vi "Process.vi"(8 "error in":errorcluster, 11 "LHF.SimpleAuth.User":refnum<class "LHF.SimpleAuth.User.lvclass">) -> (0 "error out":errorcluster={"status"=TRUE, "code"=1556, "source"="In Place Element Structure in SMO.lvclass:GetProtectedEvents.vi->SMO.lvclass:Process.vi:5310001->SMO.UI.lvclass:Process.vi:5310001->LHF.SimpleAuth.User.lvclass:Process.vi"}, 3 "LHF.SimpleAuth.User out":refnum<class "LHF.SimpleAuth.User.lvclass">)   [LabVIEW 2013, in "LHF.SimpleAuth.User.lvclass"]
doc: "---------------------------------------------------------------\nJKI State Machine Objects™\nhttp://jki.net/state-machine-objects/\nCopyright (C) 2005-2015, JKI <info@jki.net>\nALL RIGHTS RESERVEDJKI State Machine Objects (SMO) 1.0.0.5\nJKI - JKI\nCopyright (c) 2016, JKI"
uses:
  LHF.SimpleAuth.User.lvclass
  <vilib>/JKI/JKI SMO/SMO/Typedefs/Parent Call--Enum.ctl
  <vilib>/JKI/JKI SMO/SMO.UI/SMO.UI.lvclass
  <userlib>/LHF/MongoDB/LHF.DB.Mongo.lvclass
  <userlib>/_OpenG.lib/md5/md5.llb/MD5 Message Digest (Hexadecimal String)__ogtk.vi
  <vilib>/JKI/JKI SMO/SMO/SMO.lvclass
panel:
  in  "Action: Edit >> Level":T1(ring)
  in  "Action: Edit >> Name":string
  in  "Action: Edit >> Login":string
  in  "Action: Load User":i32(listbox)=-1
  in  "Action: Save":bool
  in  "Action: Set Password":bool
  in  "Action: Remove":bool
  # "For instructions on how to use the JKI State Machine Objects, examples and video tutorials, visit:\nhttp://jki.net/state-machine-objects/\n\nJKI State Machine Objects™\nhttp://jki.net/state-machine-objects/\nCopyright (C) 2005-2015, JKI <info@jki.net>\nALL RIGHTS RESERVED"
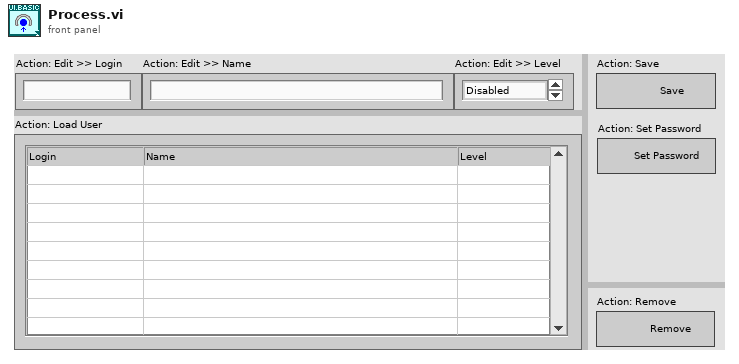
[diagram p1: front panel]
types:
  T1 = enum16{"Disabled", "Operator", "Engineer", "Administrator"}
  T2 = typedef "SMO.lvclass/Parent Call--Enum.ctl" = enum16{"Allows parent to run", "Does not request parent to run"}
  T3 = enum32{"invalid app kind", "Development System", "Run Time System", "Student Edition", "Embedded LabVIEW", "Evaluation", "Custom"}
  T4 = enum32{"Invalid", "Standard", "Closed", "Hidden", "Minimized", "Maximized"}
  T5 = enum32{"Bad", "Idle", "Run top level", "Running"}
  T6 = cluster{"login":string, "name":string, "level":u8}
  T7 = cluster{"Core":cluster{"Current VI Reference":refnum<vi>, "Close Panel on Exit?":bool, "error":errorcluster}, "Self Reference":refnum<class "LHF.SimpleAuth.User.lvclass">, "Mongo":refnum<class "LHF.DB.Mongo.lvclass">, "ObjectIDs":string[], "ObjectID":string, "User":cluster{"login":string, "name":string, "level":u8}, "Edit":cluster{"login":string, "name":string, "level":u8}}
  T8 = cluster{"Current VI Reference":refnum<vi>, "Close Panel on Exit?":bool, "error":errorcluster}
  T9 = typedef "SMO.lvclass/Protected Events.ctl" = cluster{"StopProcesses":refnum<user-event>, "AbortProcesses":refnum<user-event>}
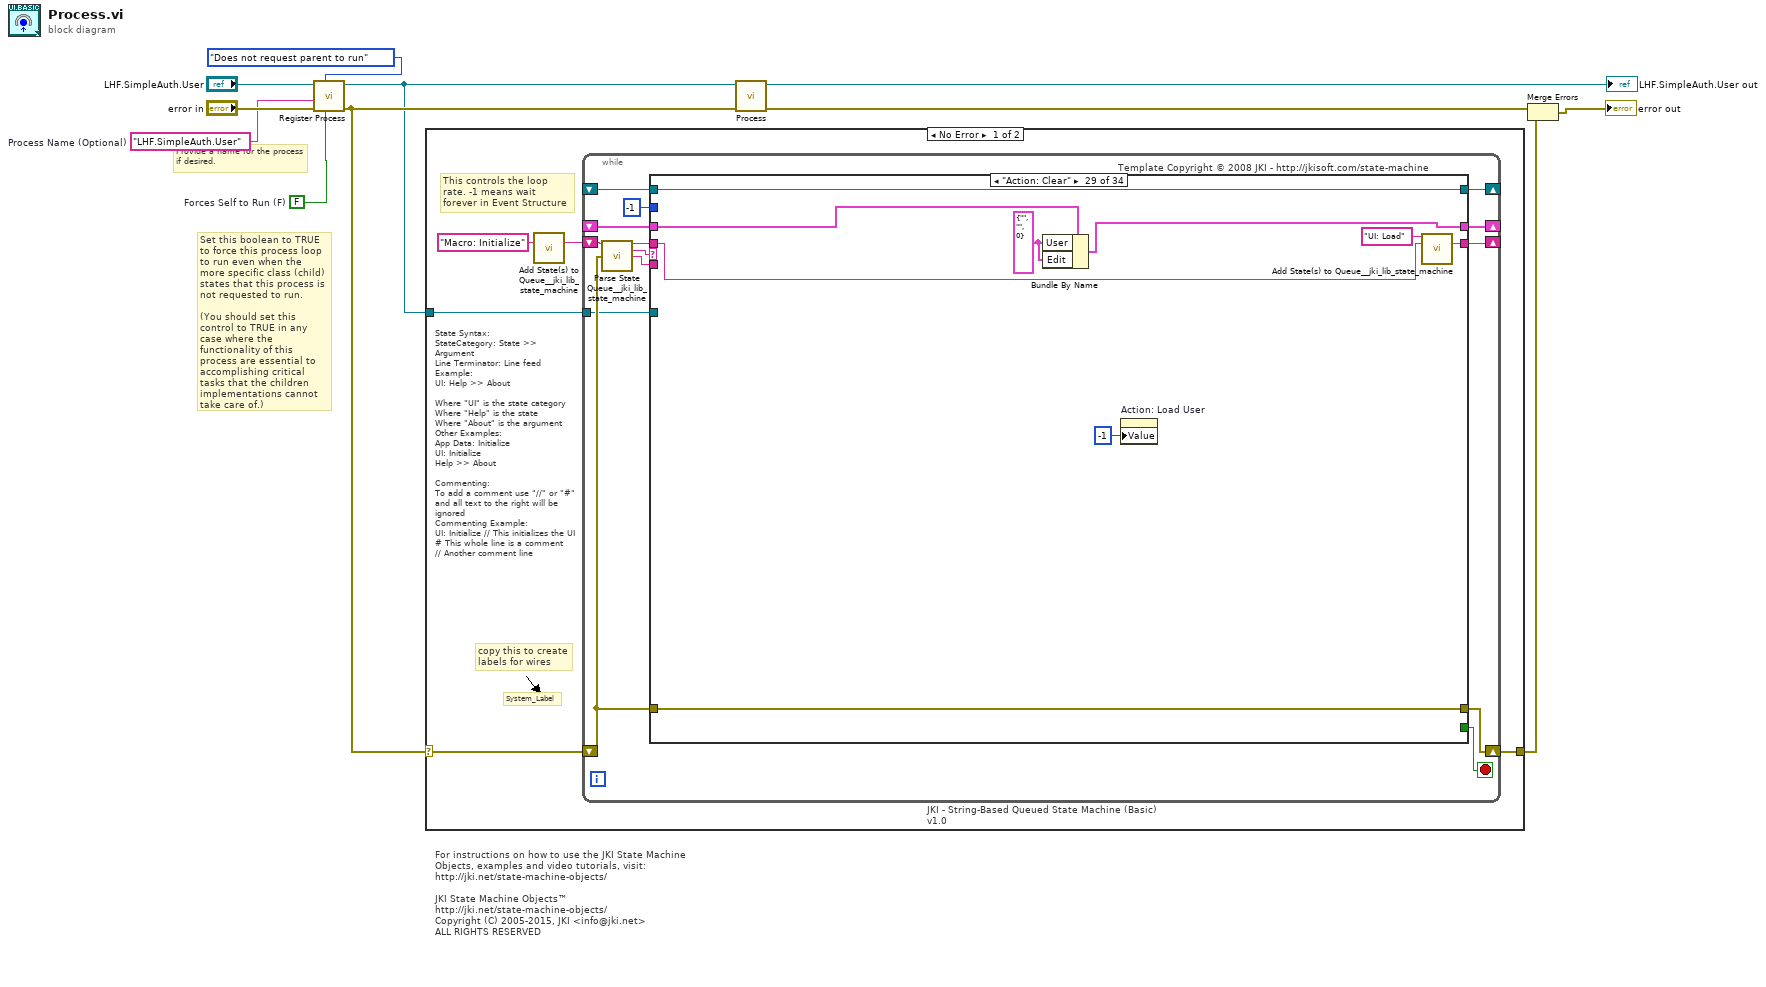
[diagram p0: block diagram]
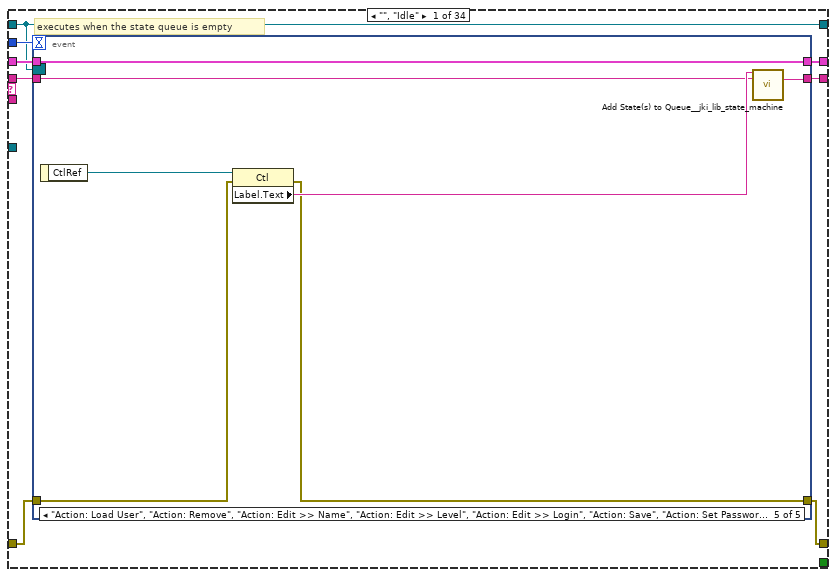
[diagram p2: hidden frame]
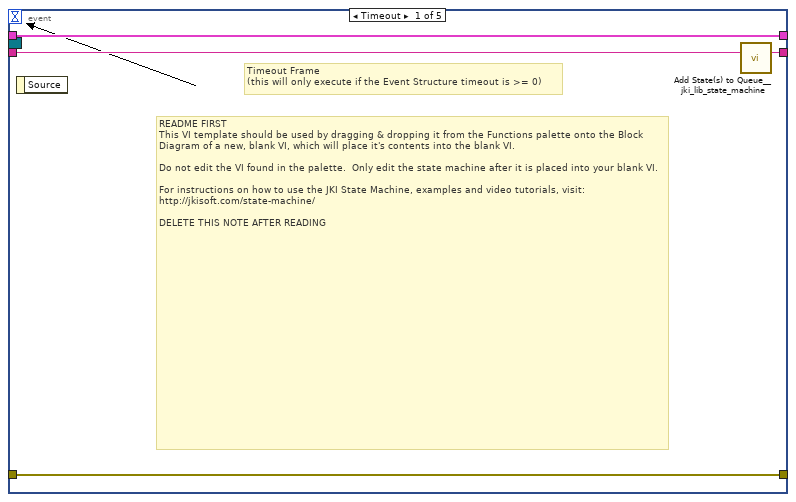
[diagram p3: hidden frame]
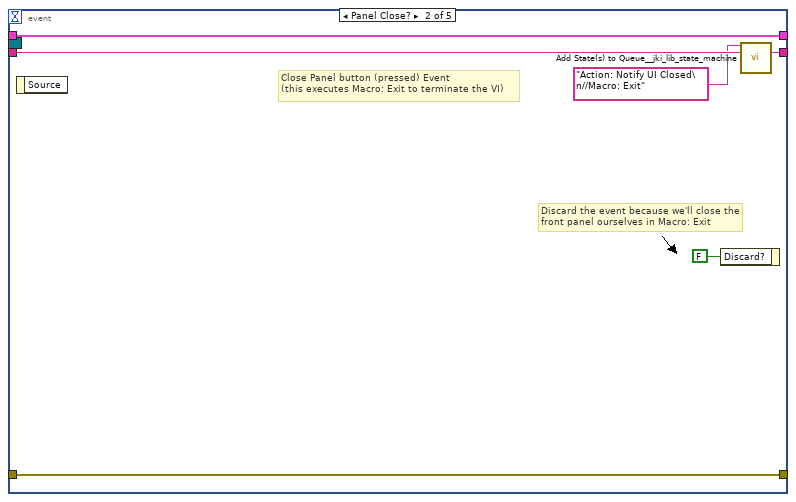
[diagram p4: hidden frame]
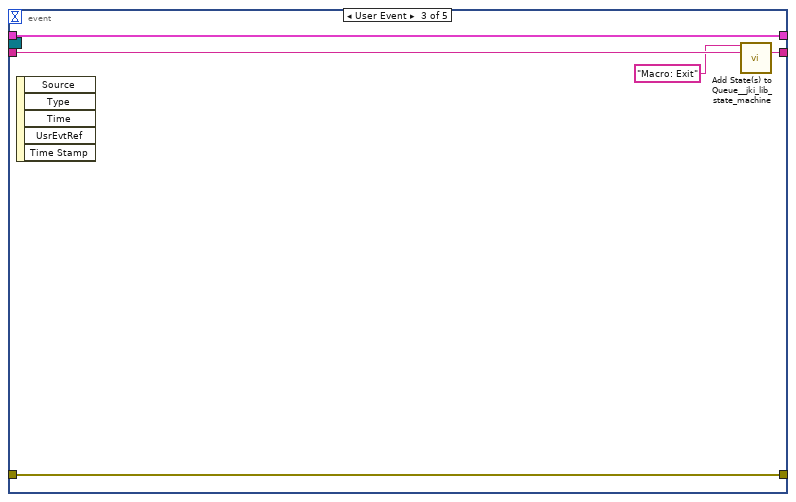
[diagram p5: hidden frame]
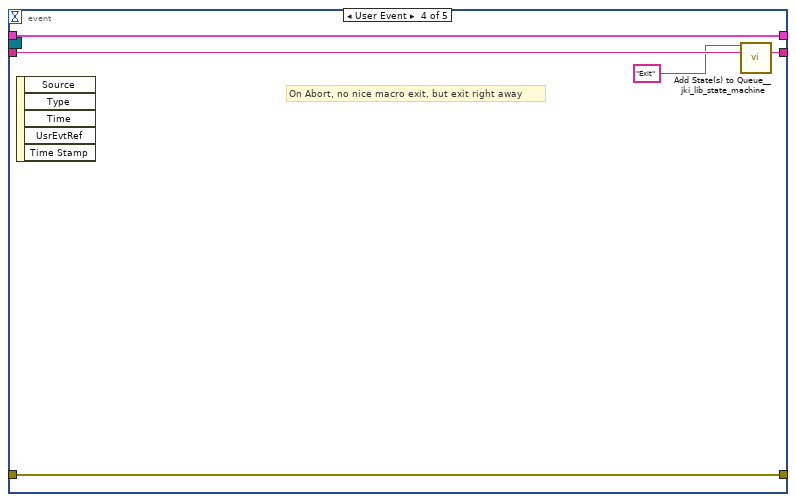
[diagram p6: hidden frame]
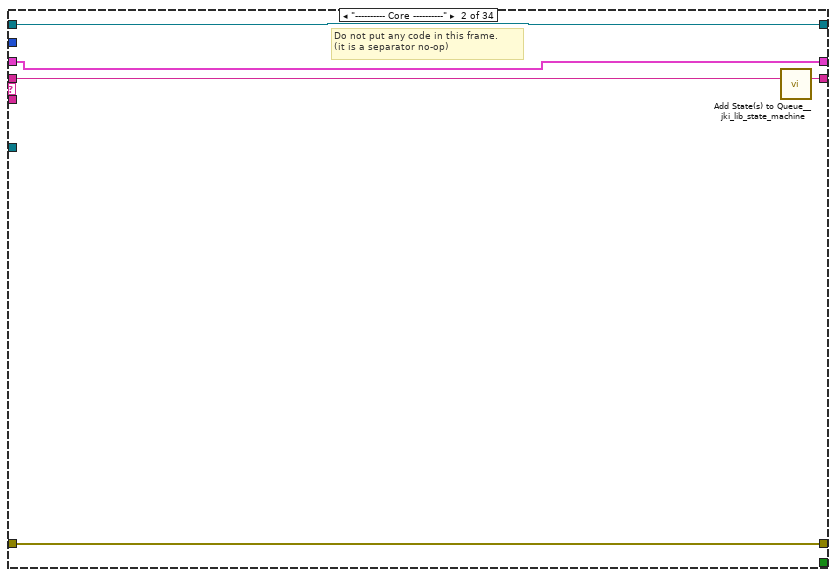
[diagram p7: hidden frame]
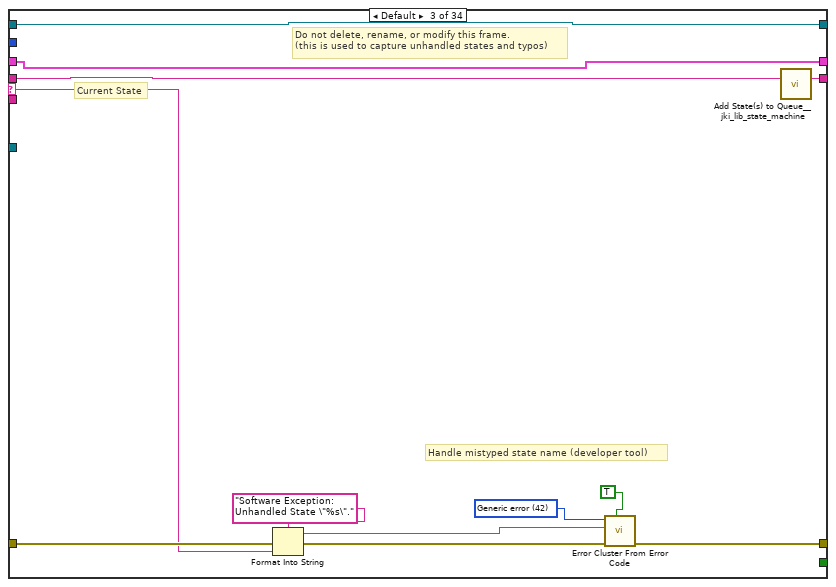
[diagram p8: hidden frame]
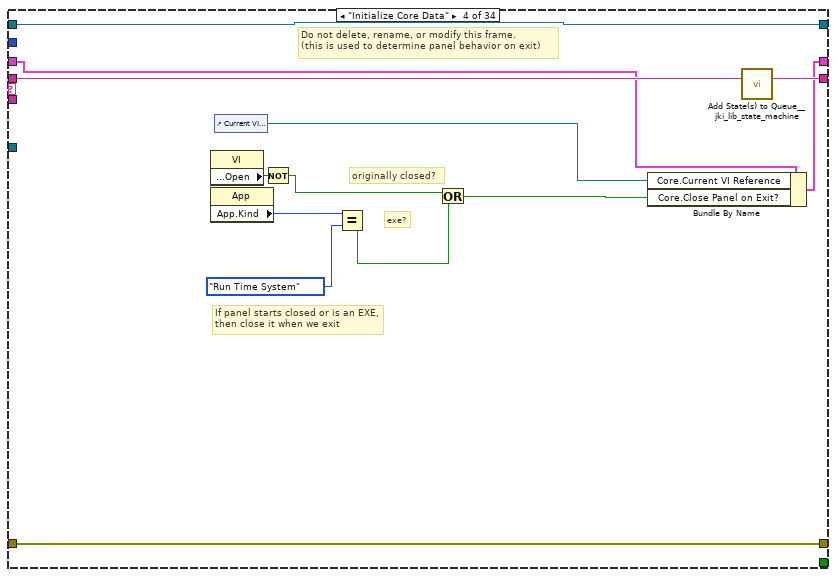
[diagram p9: hidden frame]
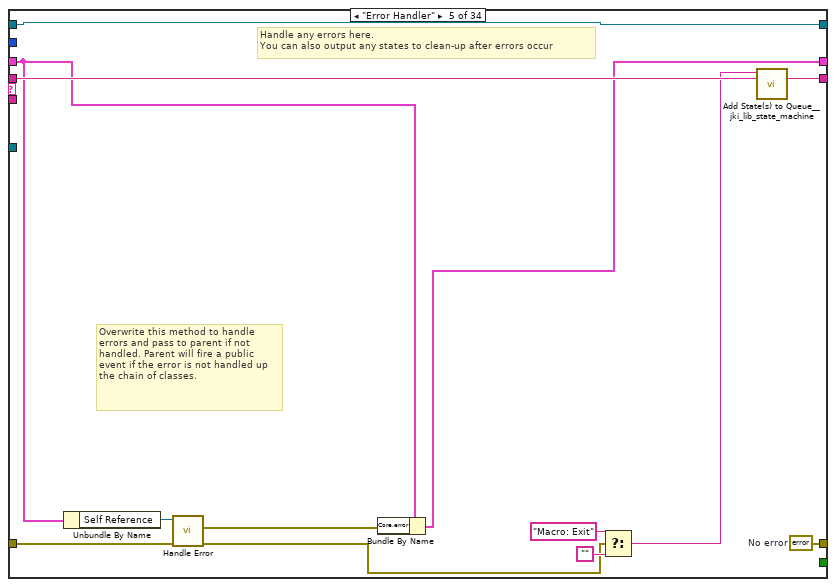
[diagram p10: hidden frame]
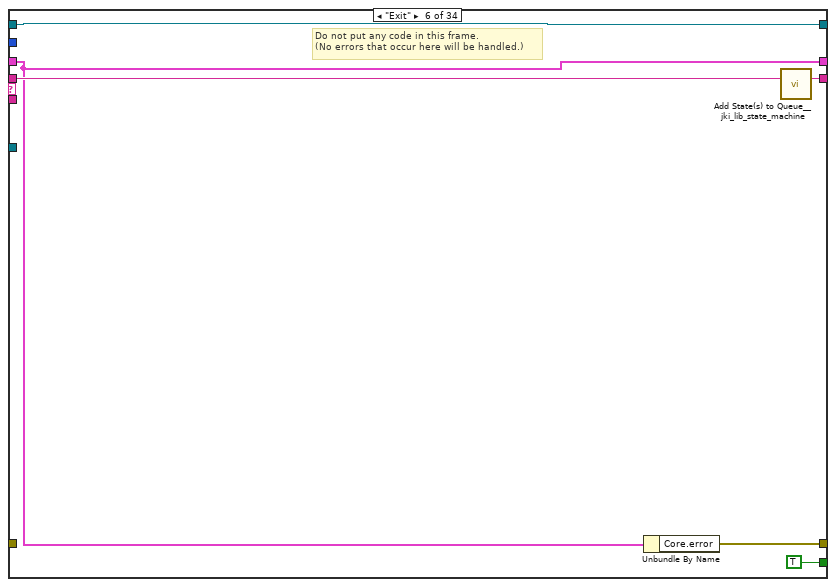
[diagram p11: hidden frame]
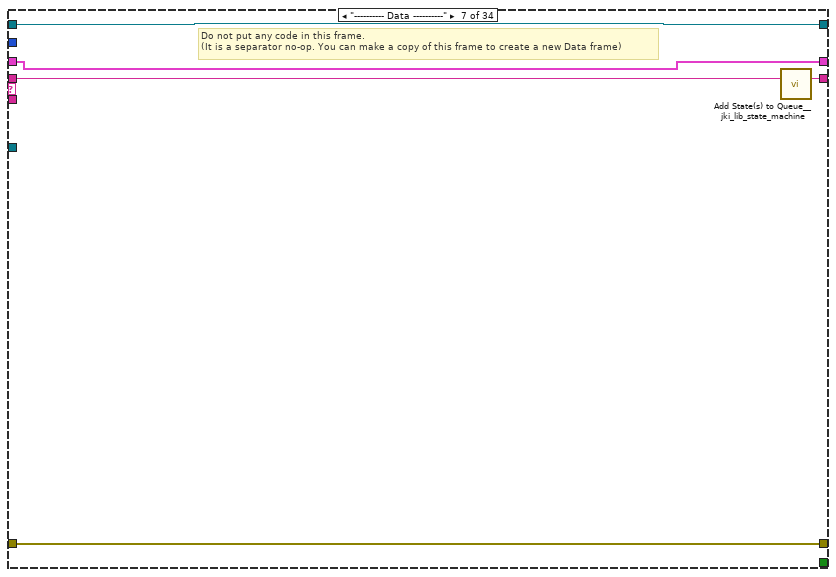
[diagram p12: hidden frame]
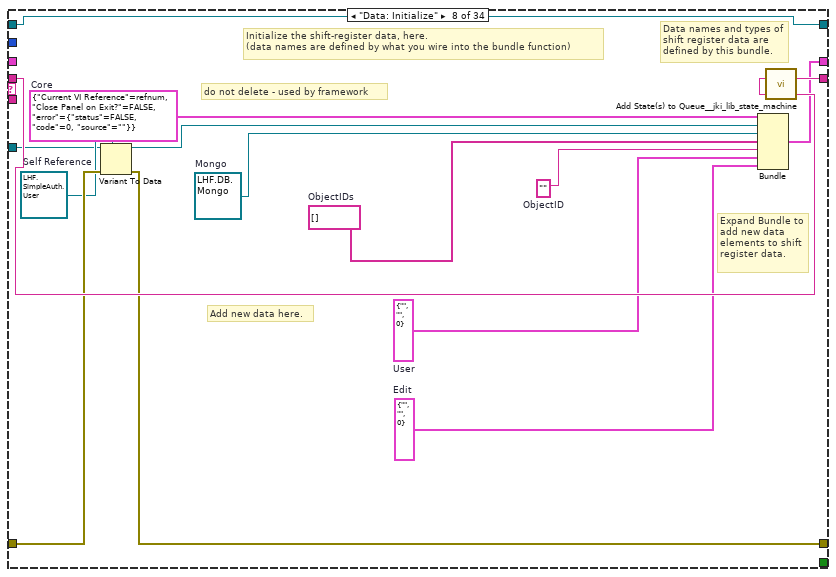
[diagram p13: hidden frame]
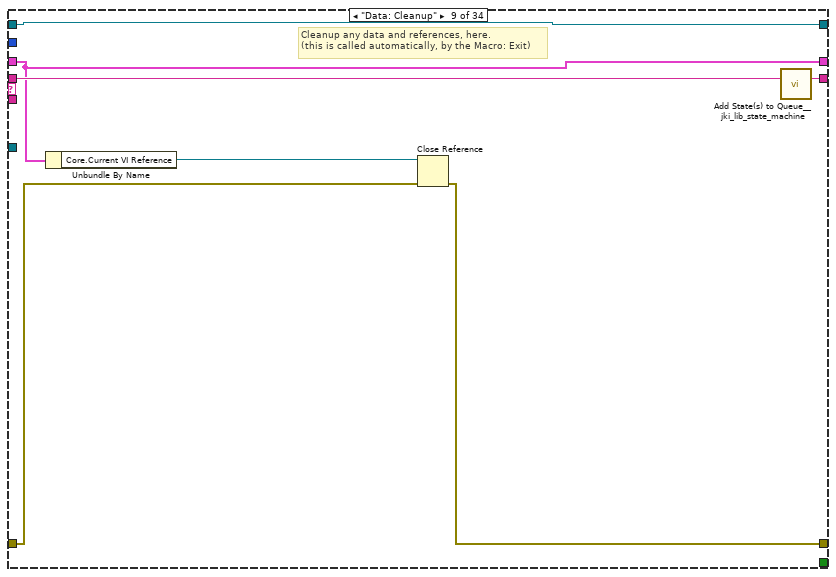
[diagram p14: hidden frame]
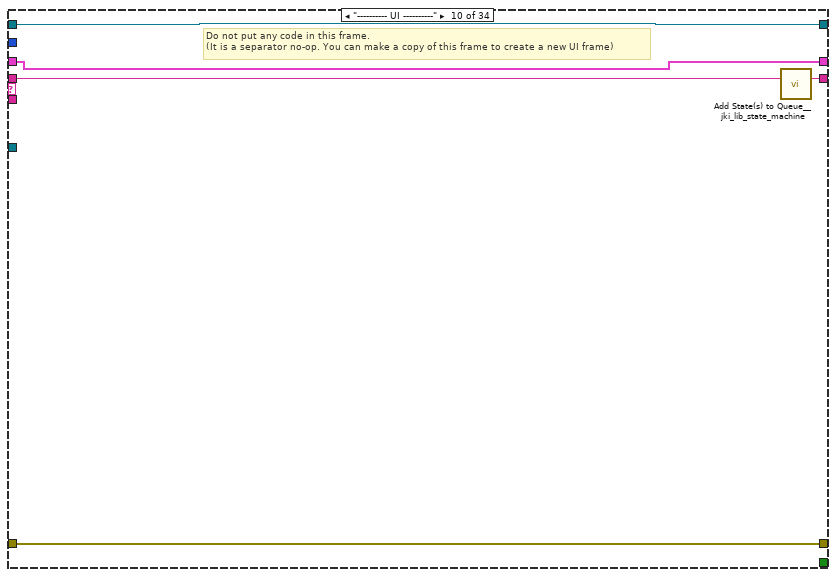
[diagram p15: hidden frame]
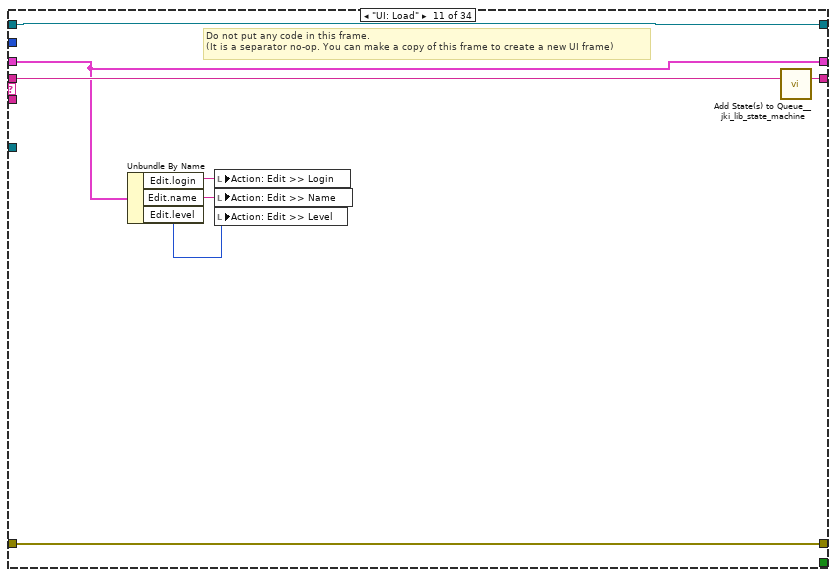
[diagram p16: hidden frame]
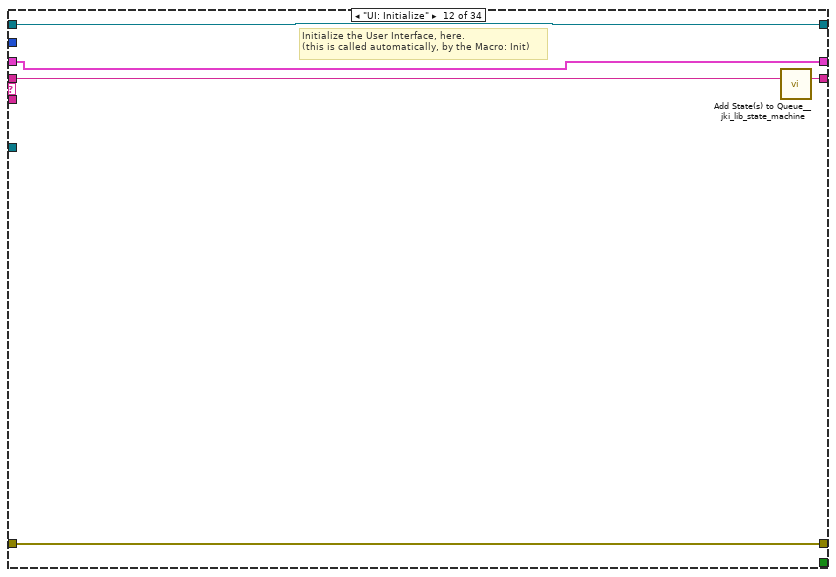
[diagram p17: hidden frame]
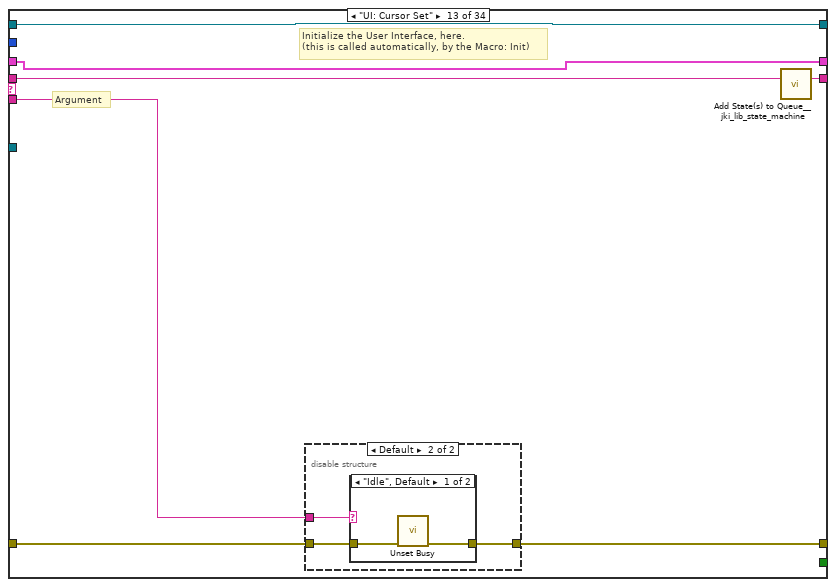
[diagram p18: hidden frame]
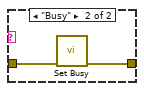
[diagram p20: hidden frame]
diagram:
  w2 = FALSE  # Forces Self to Run (F)
  w1 = "LHF.SimpleAuth.User"  # Process Name (Optional)
  # "Provide a name for the process\nif desired."
  # "Set this boolean to TRUE to force this process loop to run even when the more specific class (child) states that this process is not requested to run.\n\n(You should set this control to TRUE in any case where the functionality of this process are essential to accomplishing critical tasks that the children implementations cannot take care of.)"
  # "For instructions on how to use the JKI State Machine Objects, examples and video tutorials, visit:\nhttp://jki.net/state-machine-objects/\n\nJKI State Machine Objects™\nhttp://jki.net/state-machine-objects/\nCopyright (C) 2005-2015, JKI <info@jki.net>\nALL RIGHTS RESERVED"
  n1 = call <vilib>:"Register Process.vi"("Forces Self to Run (F)"=w2, "Parent Call"=Parent_Call--Enum."Does not request parent to run", "error in (no error)"="error in", "Process Name (optional)"=w1, "SMO"="LHF.SimpleAuth.User") -> ("error out"=w8:errorcluster, "SMO out"=w7:refnum<class "LHF.SimpleAuth.User.lvclass">)  [unwired: 5 in]
  n2 = case shown="No Error" w8 {
    selector: w8 -> [w13 w488]
    tunnel: w7 -> [w14 _]
    tunnel: [w12 w488] -> w4
    frame No Error {
      # "State Syntax:\nStateCategory: State >> Argument\nLine Terminator: Line feed\nExample:\nUI: Help >> About\n\nWhere \"UI\" is the state category\nWhere \"Help\" is the state\nWhere \"About\" is the argument\nOther Examples:\nApp Data: Initialize\nUI: Initialize\nHelp >> About\n\nCommenting:\nTo add a comment use \"//\" or \"#\" and all text to the right will be ignored\nCommenting Example:\nUI: Initialize // This initializes the UI\n# This whole line is a comment\n// Another comment line"
      # "copy this to create labels for wires"
      # "This controls the loop rate. -1 means wait forever in Event Structure"
      # "System_Label"
      n3 = call <vilib>:"Add State(s) to Queue__jki_lib_state_machine.vi"("State(s) in (\"\")"="Macro: Initialize") -> ("States Out"=w16:string)  [unwired: 14 in]
      n4 = while "JKI - String-Based Queued State Machine (Basic) v1.0" {
        shift-right: [w23] -> _
        shift-left: _ -> [w22]
        shift-right: [w26] -> w12
        shift-left: w13 -> [w20]
        shift-right: [w25] -> _
        shift-left: w16 -> [w27]
        tunnel: w14 -> [w19]
        shift-right: [w18] -> _
        shift-left: _ -> [w17]
        stop <- w24 stop-if-true
        # "Template Copyright © 2008 JKI - http://jkisoft.com/state-machine"
        n5 = call <vilib>:"Parse State Queue__jki_lib_state_machine.vi"("State Queue"=w27, "Error In (no error)"=w20) -> ("Remaining States"=w29:string, "Current State"=w30:string, "Arguments"=w28:string)  [unwired: 11 in]
        n6 = case shown="\"Action: Clear\"" w30 {
          selector: w30 -> [_ _ w72 _ _ _ _ _ _ _ _ _ _ _ _ _ _ _ _ _ _ _ _ _ _ _ _ _ _ _ _ _ _ _]
          tunnel: w29 -> [w38 w70 w76 w95 w108 w114 w119 w134 w141 w146 w154 w159 w166 w182 w214 w228 w242 w247 w258 w263 w274 w289 w294 w307 w331 w336 w346 w363 w396 w409 w418 w427 w465 w487]
          tunnel: w28 -> [_ _ _ _ _ _ _ _ _ _ _ _ w160 w176 _ _ _ _ _ _ _ _ _ _ _ _ _ _ _ _ _ _ _ _]
          tunnel: w22 -> [w36 w67 w74 w86 w97 w110 w116 _ w136 w143 w147 w157 w164 w178 w211 w224 w233 w244 w255 w260 w272 w287 w292 w304 w328 w334 w343 w360 w394 w406 w416 w424 w462 w483]
          tunnel: [w35 w68 w78 w92 w99 w109 w117 w130 w137 w144 w152 w156 w161 w179 w212 w226 w240 w245 w249 w261 w270 w284 w290 w297 w321 w332 w338 w355 w392 w398 w414 w422 w453 w481] -> w26
          tunnel: w20 -> [w34 w68 w77 w92 w104 _ w117 w131 w138 w144 w152 w156 w162 w180 w212 w226 w240 w245 w250 w261 w271 w285 w290 w298 w325 w332 w339 w356 w392 w399 w414 w423 w452 w482]
          tunnel: [w37 w69 w75 w94 w107 w113 w118 w133 w140 w145 w153 w158 w165 w181 w213 w227 w241 w246 w257 w262 w273 w288 w293 w306 w330 w335 w345 w362 w395 w408 w417 w426 w464 w486] -> w25
          tunnel: [_ _ _ _ _ TRUE _ _ _ _ _ _ _ _ _ _ _ _ _ _ _ _ _ _ _ _ _ _ _ _ _ _ _ _] -> w24
          tunnel: [w33 w67 w74 w93 w96 w110 w116 w132 w136 w143 w147 w157 w164 w178 w211 w224 w233 w244 w255 w260 w272 w287 w292 w296 w324 w334 w343 w360 w391 w406 w413 w421 w450 w483] -> w23
          tunnel: -1 ("Timeout") -> [w32 _ _ _ _ _ _ _ _ _ _ _ _ _ _ _ _ _ _ _ _ _ _ _ _ _ _ _ _ _ _ _ _ _]
          tunnel: w19 -> [_ _ _ _ _ _ _ w128 _ _ _ _ _ _ _ _ _ _ _ _ _ _ _ _ _ _ _ _ _ _ _ _ _ _]
          tunnel: [w31 w66 w71 w83 w106 w111 w115 w126 w135 w142 w151 w155 w163 w175 w210 w225 w234 w243 w256 w259 w269 w286 w291 w305 w329 w333 w344 w361 w393 w407 w415 w425 w463 w485] -> w18
          tunnel: w17 -> [w31 w66 w71 w83 w106 w111 w115 w126 w135 w142 w151 w155 w163 w175 w210 w225 w234 w243 w256 w259 w265 w286 w291 w305 w329 w333 w344 w361 w393 w407 w415 w425 w463 w485]
          frame "", "Idle" {
            # "executes when the state queue is empty"
            n7 = event shown="[4] \"Action: Load User\", \"Action: Remove\", \"Action: Edit >> Name\", \"Action: Edit >> Level\", \"Action: Edit >> Login\", \"Action: Save\", \"Action: Set Password\": Value Change" {
              selector: w31 -> [_ _ _ _ _]
              dyn-events: _ -> [_ _ _ _ _]
              timeout: w32 -> [_ _ _ _ _]
              tunnel: w38 -> [w42 w48 w53 w58 w59]
              tunnel: [w41 w47 w52 w57 w64] -> w37
              tunnel: w36 -> [w39 w44 w50 w55 w60]
              tunnel: [w40 w43 w51 w56 w61] -> w35
              tunnel: w34 -> [w40 w43 w51 w56 w62]
              tunnel: [w39 w44 w50 w55 w60] -> w33
              event Timeout {
                # "README FIRST\nThis VI template should be used by dragging & dropping it from the Functions palette onto the Block Diagram of a new, blank VI, which will place it's contents into the blank VI.\n\nDo not edit the VI found in the palette.  Only edit the state machine after it is placed into your blank VI.\n\nFor instructions on how to use the JKI State Machine, examples and video tutorials, visit:\nhttp://jkisoft.com/state-machine/\n\nDELETE THIS NOTE AFTER READING"
                # "Timeout Frame\n(this will only execute if the Event Structure timeout is >= 0)"
                n8 = event-data() -> ()  [unwired: 1 in, 1 out]
                n9 = call <vilib>:"Add State(s) to Queue__jki_lib_state_machine.vi"("State(s) in (\"\")"=w42) -> ("States Out"=w41:string)  [unwired: 14 in]
              }
              event Panel Close? {
                # "Discard the event because we'll close the front panel ourselves in Macro: Exit"
                # "Close Panel button (pressed) Event\n(this executes Macro: Exit to terminate the VI)"
                n10 = event-data() -> ()  [unwired: 1 in, 1 out]
                n11 = event-data("Discard?"=FALSE) -> ()  [unwired: 1 in, 1 out]
                n12 = call <vilib>:"Add State(s) to Queue__jki_lib_state_machine.vi"("State(s) in Front (\"\")"="Action: Notify UI Closed\n//Macro: Exit", "State(s) in (\"\")"=w48) -> ("States Out"=w47:string)  [unwired: 13 in]
              }
              event User Event {
                n13 = event-data() -> ()  [unwired: 1 in, 5 out]
                n14 = call <vilib>:"Add State(s) to Queue__jki_lib_state_machine.vi"("State(s) in Front (\"\")"="Macro: Exit", "State(s) in (\"\")"=w53) -> ("States Out"=w52:string)  [unwired: 13 in]
              }
              event User Event {
                # "On Abort, no nice macro exit, but exit right away"
                n15 = event-data() -> ()  [unwired: 1 in, 5 out]
                n16 = call <vilib>:"Add State(s) to Queue__jki_lib_state_machine.vi"("State(s) in Front (\"\")"="Exit", "State(s) in (\"\")"=w58) -> ("States Out"=w57:string)  [unwired: 13 in]
              }
              event "Action: Load User", "Action: Remove", "Action: Edit >> Name", "Action: Edit >> Level", "Action: Edit >> Login", "Action: Save", "Action: Set Password": Value Change {
                n17 = event-data() -> ("CtlRef"=w65:refnum<vi>)  [unwired: 1 in]
                n18 = property class="Ctl"(reference=w65, error in=w62) -> (error out=w61:errorcluster, "Label.Text"=w63:string)  [unwired: 1 out]
                n19 = call <vilib>:"Add State(s) to Queue__jki_lib_state_machine.vi"("State(s) in Front (\"\")"=w63, "State(s) in (\"\")"=w59) -> ("States Out"=w64:string)  [unwired: 13 in]
              }
            }
          }
          frame "---------- Core ----------" {
            # "Do not put any code in this frame.\n(it is a separator no-op)"
            n20 = call <vilib>:"Add State(s) to Queue__jki_lib_state_machine.vi"("State(s) in (\"\")"=w70) -> ("States Out"=w69:string)  [unwired: 14 in]
          }
          frame Default {
            w81 = 42 items=["No error", "Argument error", "Memory is full", "Out of zone", "End of file", "File already open", "Generic file I/O error", "File not found", "File permission error", "Disk is full", "Duplicate path", "Too many files open", "System feature not enabled", "Resource file not found", "Cannot add resource", "Resource not found", "Image not found", "Image memory error", "Pen does not exist", "Config type invalid", "Config token not found", "Config parse error", "Config memory error", "Bad external code format", "Bad external code offset", "External code not present", "Null window", "Destroy window error", "Null menu", "Print aborted", "Bad print record", "Print driver error", "Windows error during printing", "Memory error during printing", "Print dialog error", "Generic print error", "Invalid device refnum", "Device not found", "Device parameter error", "Device unit error", "Cannot open device", "Device call aborted", "Generic error", "Cancelled by user", "Object ID too low", "Object ID too high", "Object not in heap", "Unknown heap", "Unknown object (invalid DefProc)", "Unknown object (DefProc not in table)", "Message out of range", "Invalid (null) method", "Unknown message", "Manager call not supported", "Bad address", "Network operation in progress", "Network operation timed out", "Connection is busy", "Network attribute not supported", "Network error", "Address in use", "System out of memory", "Connection aborted", "Connection refused", "Not connected", "Already connected", "Connection closed", "Initialization error (interapplication manager)", "Bad occurrence", "Wait on unbound occurrence handler", "Occurrence queue overflow", "Datalog type conflict", "Unused", "Unrecognized type (interapplication manager)", "Memory corrupt", "Failed to make temporary DLL", "Old CIN version", "Drag socket not found", "Failed to load drop-object", "Failed to register OLE object", "Failed to release OLE object", "Format specifier type mismatch", "Unknown format specifier", "Too few format specifiers", "Too many format specifiers", "Scan failed", "Newer CIN version", "Error converting to variant", "Runtime menu error", "Password tampered", "Variant attribute not found", "Incompatible variant data type", "Event data is not available", "Event Store is not present", "Occurrence is not found", "Event Queue is not created", "Event info is not available", "Refnum passed is NULL", "Error retrieving Class GUID", "Error retrieving CoClass GUID", "Error retrieving TypeLib GUID.", "Bad built application magic bytes.", "Specific driver is different from the specific driver associated with the Logical Name.", "There is no session opened to the class driver.", "Max Error", "MAX - Error with config objects", "MAX - Error loading configuration", "MAX - Group not supported"]
            # "Current State"
            # "Do not delete, rename, or modify this frame.\n(this is used to capture unhandled states and typos)"
            # "Handle mistyped state name (developer tool)"
            n21 = Format Into String(format string="Software Exception: Unhandled State \"%s\"." ("message"), error in=w77, w72) -> (resulting string=w80:string, error out=w79:errorcluster)  [unwired: 1 in]
            n22 = call <vilib>:"Error Cluster From Error Code.vi"("show call chain? (False)"=TRUE, "error in (no error)"=w79, "error message (\"\")"=w80, "error code (0)"=w81) -> ("error out"=w78:errorcluster)  [unwired: 5 in]
            n23 = call <vilib>:"Add State(s) to Queue__jki_lib_state_machine.vi"("State(s) in (\"\")"=w76) -> ("States Out"=w75:string)  [unwired: 14 in]
          }
          frame "Initialize Core Data" {
            # "Do not delete, rename, or modify this frame.\n(this is used to determine panel behavior on exit)"
            # "originally closed?"
            # "exe?"
            # "If panel starts closed or is an EXE, then close it when we exit"
            n24 = property class="VI"() -> ("Front Panel.Open"=w91:bool)  [unwired: 2 in, 2 out]
            n25 = property class="App"() -> ("App.Kind"=w90:T3)  [unwired: 2 in, 2 out]
            n26 = control-ref of="Current VI Reference"() -> (w84:refnum<vi>)
            n27 = Not(x=w91) -> (.not. x?=w88:bool)
            n28 = Equal?(x=w90, y=T3."Run Time System" ("Application:Kind")) -> (x = y?=w87:bool)
            n29 = Or(x=w88, y=w87) -> (x .or. y?=w85:bool)
            n30 = Bundle By Name(cluster=w86, "Core.Current VI Reference"=w84, "Core.Close Panel on Exit?"=w85) -> (w93:T7)
            n31 = call <vilib>:"Add State(s) to Queue__jki_lib_state_machine.vi"("State(s) in (\"\")"=w95) -> ("States Out"=w94:string)  [unwired: 14 in]
          }
          frame "Error Handler" {
            w99 = errorcluster {"status"=FALSE, "code"=0, "source"=""}  # No error
            # "Overwrite this method to handle errors and pass to parent if not handled. Parent will fire a public event if the error is not handled up the chain of classes."
            # "Handle any errors here.\nYou can also output any states to clean-up after errors occur"
            n32 = Unbundle By Name(w97) -> ("Self Reference"=w105:refnum<class "LHF.SimpleAuth.User.lvclass">)
            n33 = call-dynamic "Handle Error.vi"("error in"=w104, "SMO"=w105) -> ("handling error"=w100:errorcluster, "Unhandled error"=w98:errorcluster)  [unwired: 7 in, 1 out]
            n34 = Bundle By Name(cluster=w97, "Core.error"=w98) -> (w96:T7)
            n35 = Select(t="Macro: Exit", s=w100, f="") -> (s? t:f=w101:string)
            n36 = call <vilib>:"Add State(s) to Queue__jki_lib_state_machine.vi"("State(s) in Front (\"\")"=w101, "State(s) in (\"\")"=w108) -> ("States Out"=w107:string)  [unwired: 13 in]
          }
          frame "Exit" {
            # "Do not put any code in this frame.\n(No errors that occur here will be handled.)"
            n37 = Unbundle By Name(w110) -> ("Core.error"=w109:errorcluster)
            n38 = call <vilib>:"Add State(s) to Queue__jki_lib_state_machine.vi"("State(s) in (\"\")"=w114) -> ("States Out"=w113:string)  [unwired: 14 in]
          }
          frame "---------- Data ----------" {
            # "Do not put any code in this frame.\n(It is a separator no-op. You can make a copy of this frame to create a new Data frame)"
            n39 = call <vilib>:"Add State(s) to Queue__jki_lib_state_machine.vi"("State(s) in (\"\")"=w119) -> ("States Out"=w118:string)  [unwired: 14 in]
          }
          frame "Data: Initialize" {
            w120 = ""  # ObjectID
            w121 = T6 {"login"="", "name"="", "level"=0}  # Edit
            w122 = T6 {"login"="", "name"="", "level"=0}  # User
            w123 = string[] []  # ObjectIDs
            w124 = refnum<class "LHF.DB.Mongo.lvclass"> refnum  # Mongo
            w125 = T8 {"Current VI Reference"=refnum, "Close Panel on Exit?"=FALSE, "error"={"status"=FALSE, "code"=0, "source"=""}}  # Core
            w129 = refnum<class "LHF.SimpleAuth.User.lvclass"> refnum  # Self Reference
            # "do not delete - used by framework"
            # "Expand Bundle to add new data elements to shift register data."
            # "Add new data here."
            # "Data names and types of shift register data are defined by this bundle."
            # "Initialize the shift-register data, here.\n(data names are defined by what you wire into the bundle function)"
            n40 = Variant To Data(error in=w131, type=w129, Variant=w128) -> (data=w127:refnum<class "LHF.SimpleAuth.User.lvclass">, error out=w130:errorcluster)
            n41 = Bundle("Core"=w125, "Self Reference"=w127, "Mongo"=w124, "ObjectIDs"=w123, "ObjectID"=w120, "User"=w122, "Edit"=w121) -> (w132:T7)  [unwired: 1 in]
            n42 = call <vilib>:"Add State(s) to Queue__jki_lib_state_machine.vi"("State(s) in (\"\")"=w134) -> ("States Out"=w133:string)  [unwired: 14 in]
          }
          frame "Data: Cleanup" {
            # "Cleanup any data and references, here.\n(this is called automatically, by the Macro: Exit)"
            n43 = Unbundle By Name(w136) -> ("Core.Current VI Reference"=w139:refnum<vi>)
            n44 = Close Reference(reference=w139, error in (no error)=w138) -> (error out=w137:errorcluster)
            n45 = call <vilib>:"Add State(s) to Queue__jki_lib_state_machine.vi"("State(s) in (\"\")"=w141) -> ("States Out"=w140:string)  [unwired: 14 in]
          }
          frame "---------- UI ----------" {
            # "Do not put any code in this frame.\n(It is a separator no-op. You can make a copy of this frame to create a new UI frame)"
            n46 = call <vilib>:"Add State(s) to Queue__jki_lib_state_machine.vi"("State(s) in (\"\")"=w146) -> ("States Out"=w145:string)  [unwired: 14 in]
          }
          frame "UI: Load" {
            # "Do not put any code in this frame.\n(It is a separator no-op. You can make a copy of this frame to create a new UI frame)"
            n47 = Unbundle By Name(w147) -> ("Edit.login"=w150:string, "Edit.name"=w149:string, "Edit.level"=w148:u8)
            n48 = local write "Action: Edit >> Login"(w150) -> ()
            n49 = local write "Action: Edit >> Name"(w149) -> ()
            n50 = local write "Action: Edit >> Level"(w148) -> ()
            n51 = call <vilib>:"Add State(s) to Queue__jki_lib_state_machine.vi"("State(s) in (\"\")"=w154) -> ("States Out"=w153:string)  [unwired: 14 in]
          }
          frame "UI: Initialize" {
            # "Initialize the User Interface, here.\n(this is called automatically, by the Macro: Init)"
            n52 = call <vilib>:"Add State(s) to Queue__jki_lib_state_machine.vi"("State(s) in (\"\")"=w159) -> ("States Out"=w158:string)  [unwired: 14 in]
          }
          frame "UI: Cursor Set" {
            # "Argument"
            # "Initialize the User Interface, here.\n(this is called automatically, by the Macro: Init)"
            n53 = disable-structure shown="Default" {
              disable-tunnel: w162 -> [w167 w170]
              disable-tunnel: [w167 w169] -> w161
              disable-tunnel: w160 -> [_ w168]
              frame condition #0 {
              }
              frame condition #1 (active) {
                n54 = case shown="\"Idle\", Default" w168 {
                  tunnel: w170 -> [w172 w174]
                  tunnel: [w171 w173] -> w169
                  frame "Idle", Default {
                    n55 = call <vilib>:"Unset Busy.vi"("error in (no error)"=w172) -> ("error out"=w171:errorcluster)  [unwired: 10 in]
                  }
                  frame "Busy" {
                    n56 = call <vilib>:"Set Busy.vi"("error in (no error)"=w174) -> ("error out"=w173:errorcluster)  [unwired: 9 in, 1 out]
                  }
                }
              }
            }
            n57 = call <vilib>:"Add State(s) to Queue__jki_lib_state_machine.vi"("State(s) in (\"\")"=w166) -> ("States Out"=w165:string)  [unwired: 14 in]
          }
          frame "UI: Front Panel State" {
            # "Argument"
            # "Set Front Panel Open or Closed\n(Usage: \"UI: Front Panel State >> Open|Close\")"
            n58 = Unbundle By Name(w178) -> ("Core.Current VI Reference"=w177:refnum<vi>)
            n59 = disable-structure shown="Default" {
              disable-tunnel: w180 -> [w186 w209]
              disable-tunnel: [w185 w209] -> w179
              disable-tunnel: w177 -> [w184 _]
              disable-tunnel: w176 -> [w183 _]
              frame condition #0 (active) {
                n60 = case shown="\"Close\"" w183 {
                  tunnel: w186 -> [w190 w203]
                  tunnel: [w192 w204] -> w185
                  tunnel: w184 -> [w191 w201]
                  frame "Open", Default {
                    n61 = property class="VI"(reference=w191, error in=w190) -> (reference out=w188:refnum<vi>, error out=w189:errorcluster, "FP.State"=w187:T4)
                    n62 = case shown="\"Closed\"" w187 {
                      tunnel: [w195 w198] -> w192
                      tunnel: w189 -> [w194 w198]
                      tunnel: w188 -> [w193 _]
                      frame "Closed" {
                        n63 = invoke class="VI" method="FP.Open"(reference=w193, error in=w194, "Activate"=TRUE, "State"=T4."Standard") -> (error out=w195:errorcluster)  [unwired: 1 in, 4 out]
                      }
                      frame Default {
                      }
                    }
                  }
                  frame "Close" {
                    n64 = property class="VI"(reference=w201, error in=w203) -> (reference out=w200:refnum<vi>, error out=w202:errorcluster, "FP.State"=w199:T4)
                    n65 = case shown="Default" w199 {
                      tunnel: [w205 w208] -> w204
                      tunnel: w202 -> [w205 w207]
                      tunnel: w200 -> [_ w206]
                      frame "Invalid", "Closed" {
                      }
                      frame Default {
                        n66 = invoke class="VI" method="FP.Close"(reference=w206, error in=w207) -> (error out=w208:errorcluster)  [unwired: 1 in, 2 out]
                      }
                    }
                  }
                }
              }
              frame condition #1 {
              }
            }
            n67 = call <vilib>:"Add State(s) to Queue__jki_lib_state_machine.vi"("State(s) in (\"\")"=w182) -> ("States Out"=w181:string)  [unwired: 14 in]
          }
          frame "---------- Macro ----------" {
            # "Do not put any code in this frame.\n(It is a separator no-op. You can make a copy of this frame to create a new Macro frame)"
            n68 = call <vilib>:"Add State(s) to Queue__jki_lib_state_machine.vi"("State(s) in (\"\")"=w214) -> ("States Out"=w213:string)  [unwired: 14 in]
          }
          frame "Macro: Initialize" {
            w219 = "Database: Connect\nAction: List Users\nUI: Initialize\n//UI: Front Panel State >> Open"  # Database: Connect Action: List Users UI: Initialize //UI: Front Panel State >> Open
            w215 = "Process: Sync"
            # "Initialization Macro\n(This is called once, when the VI starts)"
            n69 = control-ref of="This VI"() -> (w217:refnum<vi>)
            n70 = property class="VI"(reference=w217) -> ("Exec.State"=w216:T5)  [unwired: 1 in, 2 out]
            n71 = Equal?(x=w216, y=T5."Run top level") -> (x = y?=w222:bool)
            n72 = Select(t=w215, s=w222, f="") -> ()  [unwired: 1 out]
            n73 = call <vilib>:"Add State(s) to Queue__jki_lib_state_machine.vi"("State(s) in Front (\"\")"="Data: Initialize\nInitialize Core Data\nEvents: Register\n", "State(s) in (\"\")"=w215, "State(s) at Back (\"\")"=w219) -> ("States Out"=w218:string)  [unwired: 12 in]
            n74 = call <vilib>:"Add State(s) to Queue__jki_lib_state_machine.vi"("State(s) in Front (\"\")"=w218, "State(s) in (\"\")"=w228) -> ("States Out"=w227:string)  [unwired: 13 in]
          }
          frame "Macro: Exit" {
            # "Exit Macro\n(This is called once, when the VI exits)"
            n75 = Unbundle By Name(w233) -> ("Core.Close Panel on Exit?"=w239:bool)
            n76 = Select(t="//UI: Front Panel State >> Close", s=w239, f="") -> (s? t:f=w236:string)
            n77 = call <vilib>:"Add State(s) to Queue__jki_lib_state_machine.vi"("State(s) in Front (\"\")"="Data: Cleanup\nEvents: Unregister\nDatabase: Disconnect", "State(s) in (\"\")"="Process: Sync", "State(s) at Back (\"\")"="Exit") -> ("States Out"=w230:string)  [unwired: 12 in]
            n78 = call <vilib>:"Add State(s) to Queue__jki_lib_state_machine.vi"("State(s) in (\"\")"=w236, "State(s) at Back (\"\")"=w230) -> ("States Out"=w235:string)  [unwired: 13 in]
            n79 = call <vilib>:"Add State(s) to Queue__jki_lib_state_machine.vi"("State(s) in Front (\"\")"=w235, "State(s) in (\"\")"=w242) -> ("States Out"=w241:string)  [unwired: 13 in]
          }
          frame "---------- Process ----------" {
            # "Template Separator\n(You can make a copy of, or modify, this frame)"
            n80 = call <vilib>:"Add State(s) to Queue__jki_lib_state_machine.vi"("State(s) in (\"\")"=w247) -> ("States Out"=w246:string)  [unwired: 14 in]
          }
          frame "Process: Sync" {
            n81 = Unbundle By Name(w255) -> ("Self Reference"=w251:refnum<class "LHF.SimpleAuth.User.lvclass">)
            n82 = call <vilib>:"WaitOnProcessSync.vi"("error in (no error)"=w250, "SMO"=w251) -> ("error out"=w249:errorcluster, "Don't run?"=w254:bool)  [unwired: 7 in, 1 out]
            n83 = Select(t="Data: Cleanup\nEvents: Unregister\nExit", s=w254, f="") -> (s? t:f=w248:string)
            n84 = call <vilib>:"Add State(s) to Queue__jki_lib_state_machine.vi"("State(s) in Front (\"\")"=w248, "State(s) in (\"\")"=w258) -> ("States Out"=w257:string)  [unwired: 13 in]
          }
          frame "---------- Events ----------" {
            # "Template Separator\n(You can make a copy of, or modify, this frame)"
            n85 = call <vilib>:"Add State(s) to Queue__jki_lib_state_machine.vi"("State(s) in (\"\")"=w263) -> ("States Out"=w262:string)  [unwired: 14 in]
          }
          frame "Events: Register" {
            # "Self Events (API Calls)"
            # "Base Class Protected Events"
            n86 = Unbundle By Name(w272) -> ("Self Reference"=w267:refnum<class "LHF.SimpleAuth.User.lvclass">)
            n87 = call <vilib>:"GetProtectedEvents.vi"("error in (no error)"=w271, "SMO"=w267) -> ("error out"=w264:errorcluster, "SMO Protected Events"=w268:T9)  [unwired: 7 in, 1 out]
            n88 = Not A Number/Path/Refnum?(number/path/refnum=w265) -> (NaN/Path/Refnum?=w266:bool)
            n89 = case shown="False" w266 {
              tunnel: [w278 w283] -> w270
              tunnel: [w277 w282] -> w269
              tunnel: w268 -> [w276 w281]
              tunnel: w264 -> [w275 w280]
              tunnel: w265 -> [_ w279]
              frame True {
                # "Expand to add\nmore events"
                n90 = register-events(error in=w275, w276) -> (reference out=w277:refnum<event-registration>, error out=w278:errorcluster)  [unwired: 1 in]
              }
              frame False {
                n91 = register-events(reference=w279, error in=w280, w281) -> (reference out=w282:refnum<event-registration>, error out=w283:errorcluster)
              }
            }
            n92 = call <vilib>:"Add State(s) to Queue__jki_lib_state_machine.vi"("State(s) in (\"\")"=w274) -> ("States Out"=w273:string)  [unwired: 14 in]
          }
          frame "Events: Unregister" {
            n93 = Unregister For Events(event registration refnum=w286, error in=w285) -> (error out=w284:errorcluster)
            n94 = call <vilib>:"Add State(s) to Queue__jki_lib_state_machine.vi"("State(s) in (\"\")"=w289) -> ("States Out"=w288:string)  [unwired: 14 in]
          }
          frame "---------- API ----------" {
            n95 = call <vilib>:"Add State(s) to Queue__jki_lib_state_machine.vi"("State(s) in (\"\")"=w294) -> ("States Out"=w293:string)  [unwired: 14 in]
          }
          frame "Database: Connect" {
            w299 = "Example" ("database")
            w300 = "mongodb://localhost/" ("url")
            n96 = Unbundle By Name(w304) -> ("Mongo"=w303:refnum<class "LHF.DB.Mongo.lvclass">)
            n97 = call-dynamic "LHF.DB.Mongo.Client.Connect.vi"("error in (no error)"=w298, "database"=w299, "url"=w300, "LHF.DB.Mongo in"=w303) -> ("error out"=w301:errorcluster, "LHF.DB.Mongo out"=w302:refnum<class "LHF.DB.Mongo.lvclass">)  [unwired: 6 in]
            n98 = case shown="Error" w301 {
              selector: w301 -> [w308 _]
              tunnel: w302 -> [w309 w319]
              tunnel: w300 -> [_ w317]
              tunnel: w299 -> [_ w316]
              tunnel: [w309 w314] -> w295
              tunnel: [w308 w313] -> w297
              frame No Error {
              }
              frame Error {
                n99 = call <vilib>:"Application Directory.vi"() -> ("Application Directory"=w312:path)
                n100 = Build Path(base path=w312, name or relative path="data\\db") -> (appended path=w311:path)
                n101 = call-dynamic "LHF.DB.Mongo.Daemon.Start.vi"("data folder"=w311, "mongod path"=path "C:/Program Files/MongoDB/Server/3.2/bin/mongod.exe", "LHF.DB.Mongo in"=w319) -> ("error out"=w315:errorcluster, "LHF.DB.Mongo out"=w318:refnum<class "LHF.DB.Mongo.lvclass">)  [unwired: 7 in]
                n102 = call-dynamic "LHF.DB.Mongo.Client.Connect.vi"("error in (no error)"=w315, "database"=w316, "url"=w317, "LHF.DB.Mongo in"=w318) -> ("error out"=w313:errorcluster, "LHF.DB.Mongo out"=w314:refnum<class "LHF.DB.Mongo.lvclass">)  [unwired: 6 in]
              }
            }
            n103 = Bundle By Name(cluster=w304, "Mongo"=w295) -> (w296:T7)
            n104 = call <vilib>:"Add State(s) to Queue__jki_lib_state_machine.vi"("State(s) in (\"\")"=w307) -> ("States Out"=w306:string)  [unwired: 14 in]
          }
          frame "Database: Disconnect" {
            n105 = Unbundle By Name(w328) -> ("Mongo"=w327:refnum<class "LHF.DB.Mongo.lvclass">)
            n106 = call-dynamic "LHF.DB.Mongo.Client.Disconnect.vi"("error in (no error)"=w325, "LHF.DB.Mongo in"=w327) -> ("error out"=w321:errorcluster, "LHF.DB.Mongo out"=w326:refnum<class "LHF.DB.Mongo.lvclass">)  [unwired: 8 in]
            n107 = call-dynamic "LHF.DB.Mongo.Daemon.Shutdown.vi"("error in (no error)"=w321, "LHF.DB.Mongo in"=w326) -> ("error out"=w323:errorcluster, "LHF.DB.Mongo out"=w322:refnum<class "LHF.DB.Mongo.lvclass">)  [unwired: 8 in]
            n108 = call <vilib>:"Clear Errors.vi"("error in (no error)"=w323) -> ()  [unwired: 6 in, 1 out]
            n109 = Bundle By Name(cluster=w328, "Mongo"=w322) -> (w324:T7)
            n110 = call <vilib>:"Add State(s) to Queue__jki_lib_state_machine.vi"("State(s) in (\"\")"=w331) -> ("States Out"=w330:string)  [unwired: 14 in]
          }
          frame "---------- Action ----------" {
            n111 = call <vilib>:"Add State(s) to Queue__jki_lib_state_machine.vi"("State(s) in (\"\")"=w336) -> ("States Out"=w335:string)  [unwired: 14 in]
          }
          frame "Action: Remove" {
            n112 = local read "Action: Load User"() -> (w342:i32)
            n113 = Unbundle By Name(w343) -> ("Mongo"=w340:refnum<class "LHF.DB.Mongo.lvclass">, "ObjectIDs"=w341:string[])
            n114 = case shown="0.." w342 {
              selector: w342 -> [_ w353]
              tunnel: w341 -> [_ w354]
              tunnel: w340 -> [_ w352]
              tunnel: w339 -> [w347 w349]
              tunnel: [w347 w348] -> w338
              frame Default {
              }
              frame 0.. {
                n115 = Index Array(array=w354, index=w353) -> (element=w350:string)
                n116 = call-dynamic "LHF.DB.Mongo.Collection.Remove.vi"("ObjectID"=w350, "error in (no error)"=w349, "collectionName"="User", "LHF.DB.Mongo in"=w352) -> ("error out"=w348:errorcluster)  [unwired: 6 in, 1 out]
              }
            }
            n117 = call <vilib>:"Add State(s) to Queue__jki_lib_state_machine.vi"("State(s) in Front (\"\")"="Action: Clear\nAction: List Users" ("State(s) in Front (\"\")"), "State(s) in (\"\")"=w346) -> ("States Out"=w345:string)  [unwired: 13 in]
          }
          frame "Action: Set Password" {
            n118 = local read "Action: Load User"() -> (w358:i32)
            n119 = Unbundle By Name(w360) -> ("Mongo"=w357:refnum<class "LHF.DB.Mongo.lvclass">, "ObjectIDs"=w359:string[])
            n120 = case shown="0.." w358 {
              selector: w358 -> [_ w371]
              tunnel: w359 -> [_ w373]
              tunnel: w357 -> [_ w369]
              tunnel: w356 -> [w364 w366]
              tunnel: [w364 w365] -> w355
              frame Default {
              }
              frame 0.. {
                n121 = call "Prompt User for Input"("error in (no error)"=w366) -> ("Password"=w370:string, "OK"=w372:bool, "error out"=w367:errorcluster)  [unwired: 16 in]
                n122 = Index Array(array=w373, index=w371) -> (element=w368:string)
                n123 = case shown="True" w372 {
                  tunnel: w370 -> [_ w384]
                  tunnel: w369 -> [_ w382]
                  tunnel: w368 -> [_ w379]
                  tunnel: w367 -> [w374 w378]
                  tunnel: [w374 w377] -> w365
                  frame False {
                  }
                  frame True {
                    w375 = "\"" ("string")
                    n124 = call-poly <userlib>:"MD5 Message Digest__ogtk.vi"("Message"=w384) -> ("MD5 Message Digest"=w383:string)
                    n125 = Bundle By Name(cluster=cluster{"Name":string, "JSON Value":string} {"Name"="_id", "JSON Value"=""} ("Query"), "JSON Value"=w379) -> (w380:cluster{"Name":string, "JSON Value":string})
                    n126 = Concatenate Strings(w375, w383, w375) -> (w376:string)
                    n127 = Bundle By Name(cluster=cluster{"Name":string, "JSON Value":string} {"Name"="pass", "JSON Value"=""} ("Update"), "JSON Value"=w376) -> (w385:cluster{"Name":string, "JSON Value":string})
                    n128 = call-dynamic "LHF.DB.Mongo.Collection.Update.Set.vi"("Query"=w380, "error in (no error)"=w378, "Update"=w385, "Collection"="User", "LHF.DB.Mongo in"=w382) -> ("error out"=w377:errorcluster)  [unwired: 5 in, 1 out]
                  }
                }
              }
            }
            n129 = call <vilib>:"Add State(s) to Queue__jki_lib_state_machine.vi"("State(s) in (\"\")"=w363) -> ("States Out"=w362:string)  [unwired: 14 in]
          }
          frame "Action: Clear" {
            w390 = T6 {"login"="", "name"="", "level"=0} ("User")
            n130 = Bundle By Name(cluster=w394, "User"=w390, "Edit"=w390) -> (w391:T7)
            n131 = property on="Action: Load User" class="MCListbox (strict)"("Value"=-1 ("Action: Load User")) -> ()  [unwired: 2 in, 2 out]
            n132 = call <vilib>:"Add State(s) to Queue__jki_lib_state_machine.vi"("State(s) in Front (\"\")"="UI: Load" ("State(s) in Front (\"\")"), "State(s) in (\"\")"=w396) -> ("States Out"=w395:string)  [unwired: 13 in]
          }
          frame "Action: Save" {
            n133 = Unbundle By Name(w406) -> ("Mongo"=w400:refnum<class "LHF.DB.Mongo.lvclass">, "ObjectID"=w402:string, "Edit"=w405:T6)
            n134 = Flatten To JSON(anything=w405, error in (no error)=w399) -> (JSON string=w404:string, 11:w403:errorcluster)  [unwired: 1 in]
            n135 = call-dynamic "LHF.DB.Mongo.Collection.Insert.vi"("ObjectID"=w402, "error in (no error)"=w403, "JSON Document"=w404, "Collection"="User", "LHF.DB.Mongo"=w400) -> ("error out"=w398:errorcluster)  [unwired: 3 in, 3 out]
            n136 = call <vilib>:"Add State(s) to Queue__jki_lib_state_machine.vi"("State(s) in Front (\"\")"="Action: Clear\nAction: List Users" ("State(s) at Back (\"\")"), "State(s) in (\"\")"=w409) -> ("States Out"=w408:string)  [unwired: 13 in]
          }
          frame "Action: Edit" {
            n137 = Bundle By Name(cluster=w416, "Edit.login"="Action: Edit >> Login", "Edit.name"="Action: Edit >> Name", "Edit.level"="Action: Edit >> Level") -> (w413:T7)
            n138 = call <vilib>:"Add State(s) to Queue__jki_lib_state_machine.vi"("State(s) in (\"\")"=w418) -> ("States Out"=w417:string)  [unwired: 14 in]
          }
          frame "Action: Load User" {
            n139 = case shown="0.." "Action: Load User" {
              selector: "Action: Load User" -> [_ w437]
              tunnel: w424 -> [w430 w448]
              tunnel: w423 -> [w428 w441]
              tunnel: [w428 w433] -> w422
              tunnel: [w430 w439] -> w421
              tunnel: ["Action: Clear" "UI: Load"] -> w419
              frame ..-1 {
              }
              frame 0.. {
                n140 = Unbundle By Name(w448) -> ("User"=w434:T6, "ObjectIDs"=w436:string[], "Mongo"=w447:refnum<class "LHF.DB.Mongo.lvclass">)
                n141 = Index Array(array=w436, index=w437) -> (element=w446:string)
                n142 = call-dynamic "LHF.DB.Mongo.Util.GetDocumentPart.vi"("Extract ObjectID"=TRUE, "ObjectID"=w446, "error in (no error)"=w441, "fields"=string[] ["login", "name", "level"], "Collection"="User", "LHF.DB.Mongo in"=w447) -> ("error out"=w442:errorcluster, "Document"=w443:string, "ObjectID"=w431:string)  [unwired: 2 in, 1 out]
                n143 = Unflatten From JSON(JSON string=w443, type and defaults=w434, error in (no error)=w442) -> (value=w438:T6, error out=w440:errorcluster)  [unwired: 4 in]
                n144 = Bundle By Name(cluster=w448, "ObjectID"=w431, "User"=w438, "Edit"=w438) -> (w439:T7)
                n145 = call <vilib>:"Clear Errors.vi"("error in (no error)"=w440) -> ("error out"=w433:errorcluster)  [unwired: 6 in]
              }
            }
            n146 = call <vilib>:"Add State(s) to Queue__jki_lib_state_machine.vi"("State(s) in Front (\"\")"=w419, "State(s) in (\"\")"=w427) -> ("States Out"=w426:string)  [unwired: 13 in]
          }
          frame "Action: List Users" {
            n147 = Unbundle By Name(w462) -> ("Mongo"=w461:refnum<class "LHF.DB.Mongo.lvclass">)
            n148 = call-dynamic "LHF.DB.Mongo.Util.ListCollection.vi"("error in (no error)"=w452, "fields"=string[] ["login", "name", "level"], "Collection"="User", "LHF.DB.Mongo in"=w461) -> ("error out"=w454:errorcluster, "Documents"=w459:string[], "ObjectIDs"=w449:string[])  [unwired: 4 in, 1 out]
            n149 = Bundle By Name(cluster=w462, "ObjectIDs"=w449) -> (w450:T7)
            n150 = local read "Action: Edit >> Level"() -> (w458:T1)
            n151 = for {
              tunnel: w459 -> [w480] mode=indexing
              tunnel: w458 -> [w474]
              tunnel: [w469] -> w457 mode=indexing
              tunnel: [w468] -> w456 mode=indexing
              tunnel: w454 -> [w466]
              n152 = Unflatten From JSON(JSON string=w480, type and defaults=T6 {"login"="", "name"="", "level"=0} ("cluster"), error in (no error)=w466) -> (value=w478:T6, error out=w467:errorcluster)  [unwired: 4 in]
              n153 = Unbundle(w478) -> ("login"=w477:string, "name"=w476:string, "level"=w475:u8)
              n154 = Variant To Data(error in=w467, type=w474, Variant=w475) -> (data=w472:T1, error out=w473:errorcluster)
              n155 = Format Into String(format string="%s", error in=w473, w472) -> (resulting string=w470:string, error out=w468:errorcluster)  [unwired: 1 in]
              n156 = Build Array(w477, w476, w470) -> (w469:string[])
            }
            n157 = Merge Errors(w454, w456) -> (w455:errorcluster)
            n158 = property on="Action: Load User" class="MCListbox (strict)"(error in=w455, "ItemNames"=w457) -> (error out=w453:errorcluster)  [unwired: 1 in, 1 out]
            n159 = call <vilib>:"Add State(s) to Queue__jki_lib_state_machine.vi"("State(s) in (\"\")"=w465) -> ("States Out"=w464:string)  [unwired: 14 in]
          }
          frame "Action: Notify UI Closed" {
            # "Notify that the UI has been closed"
            n160 = Unbundle By Name(w483) -> ("Self Reference"=w484:refnum<class "LHF.SimpleAuth.User.lvclass">)
            n161 = call <vilib>:"Hide.vi"("error in (no error)"=w482, "SMO.UI"=w484) -> ("error out"=w481:errorcluster)  [unwired: 8 in, 1 out]
            n162 = call <vilib>:"Add State(s) to Queue__jki_lib_state_machine.vi"("State(s) in (\"\")"=w487) -> ("States Out"=w486:string)  [unwired: 14 in]
          }
        }
      }
    }
    frame Error {
    }
  }
  n163 = call-parent "Process.vi"("error in (no error)"=w8, "SMO.UI"=w7) -> ("error out"=w5:errorcluster, "SMO.UI out"=→"LHF.SimpleAuth.User out":refnum<class "LHF.SimpleAuth.User.lvclass">)  [unwired: 8 in]
  n164 = Merge Errors(w5, w4) -> (→"error out":errorcluster)
